vi "fmeasure Test.vi"() -> ()   [LabVIEW 2018, in "Bronkhorst M14 Flow Meter.lvlib"]
uses:
  Bronkhorst M14 Flow Meter.lvlib
  Settings Cluster.ctl
panel:
  out "*(type *) &x 2":dbl
  in  "stop":bool
  out "read buffer":string
  out "Connection Error":bool
  out "*(type *) &x":dbl
  out "submatch 1":string
  out "flow":dbl
  in  "error in (no error)":errorcluster
  out "error out":errorcluster
  in  "Bronkhorst Settings in":T1
  out "Bronkhorst Settings out":T1
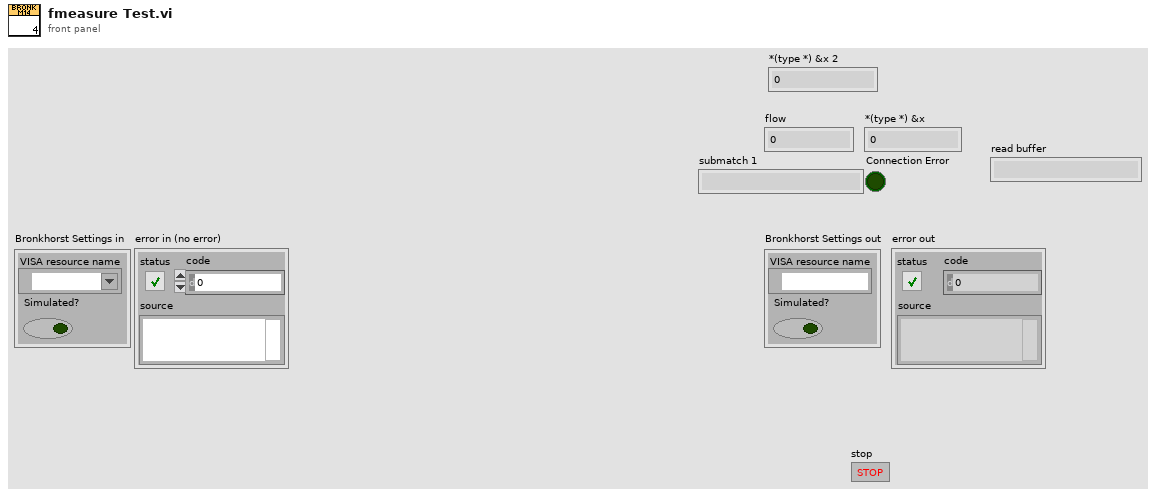
[diagram p1: front panel]
types:
  T1 = typedef "Bronkhorst M14 Flow Meter.lvlib/Settings Cluster.ctl" = cluster{"VISA resource name":refnum<visa-resource-name>, "Simulated?":bool}
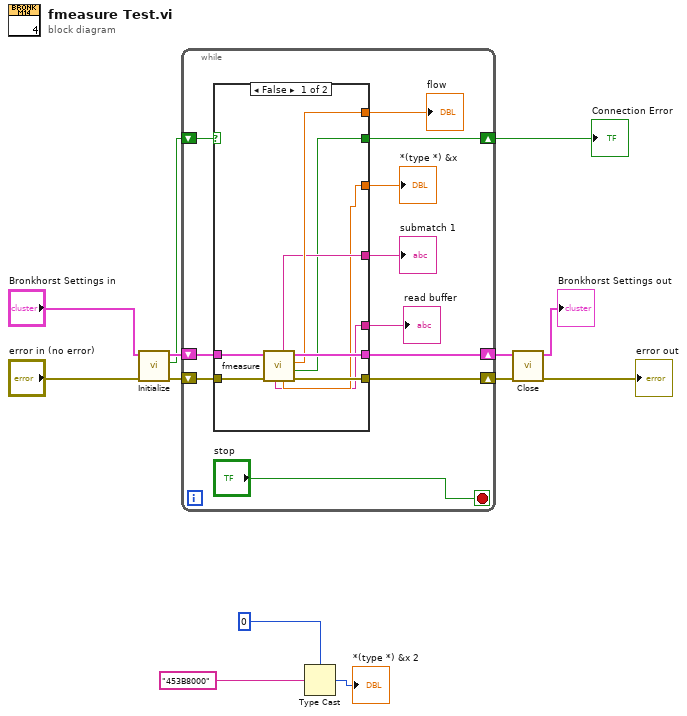
[diagram p0: block diagram]
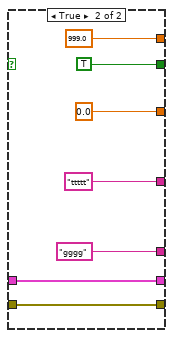
[diagram p2: hidden frame]
diagram:
  n1 = call "Initialize.vi"("error in (no error)"="error in (no error)", "Bronkhorst Settings in"="Bronkhorst Settings in") -> ("error out"=w11:errorcluster, "No Meter Connected"=w6:bool, "Bronkhorst Settings out"=w12:T1)  [unwired: 7 in]
  n2 = while {
    shift-right: [w22] -> w10
    shift-left: w12 -> [w24]
    shift-right: [w21] -> w8
    shift-left: w11 -> [w23]
    shift-right: [w19] -> w4
    shift-left: w6 -> [w20]
    stop <- "stop" stop-if-true
    n3 = case shown="False" w20 {
      tunnel: w24 -> [w33 w40]
      tunnel: w23 -> [w32 w39]
      tunnel: [w31 w40] -> w22
      tunnel: [w30 w39] -> w21
      tunnel: [w29 999.0 ("flow")] -> w14
      tunnel: [w28 "ttttt" ("submatch 1")] -> w15
      tunnel: [w27 0.0 ("*(type *) &x")] -> w16
      tunnel: [w26 TRUE ("Connection Error")] -> w19
      tunnel: [w25 "gggg" ("read buffer")] -> w17
      frame False {
        n4 = call "fmeasure.vi"("error in (no error)"=w32, "Bronkhorst Settings in"=w33) -> ("error out"=w30:errorcluster, "Connection Error"=w26:bool, "flow"=w29:dbl, "Bronkhorst Settings out"=w31:T1, "*(type *) &x"=w27:dbl, "submatch 1"=w28:string, "read buffer"=w25:string)  [unwired: 3 in]
      }
      frame True {
      }
    }
    "flow" <- w14
    "submatch 1" <- w15
    "*(type *) &x" <- w16
    "read buffer" <- w17
  }
  "Connection Error" <- w4
  n5 = Type Cast(type=0, x="453B8000") -> (*(type *) &x=→"*(type *) &x 2":i32)
  n6 = call "Close.vi"("error in (no error)"=w8, "Bronkhorst Settings in"=w10) -> ("error out"=→"error out":errorcluster, "Bronkhorst Settings out"=→"Bronkhorst Settings out":T1)  [unwired: 8 in]
